vi "Receive Telemetry Packet.vi"(11 "UDP Network Connection in":refnum<k16>) -> (2 "Telemetry Packet":T1)   [LabVIEW 2015]
uses:
  Telemetry Packet Type.ctl
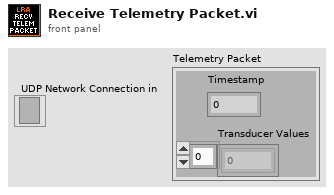
[diagram p1: front panel]
types:
  T1 = typedef "Telemetry Packet Type.ctl" = cluster{"Timestamp\n":u32, "Transducer Values":dbl[]}
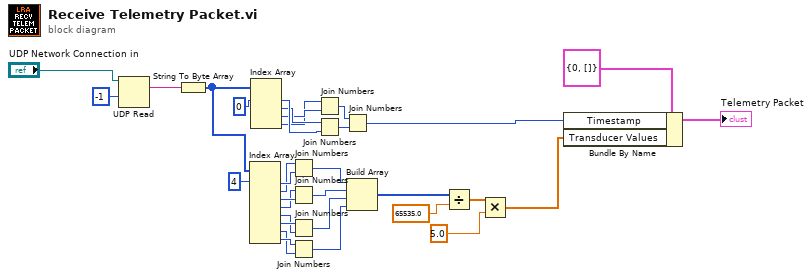
[diagram p0: block diagram]
diagram:
  n1 = UDP Read(connection ID="UDP Network Connection in", timeout ms (25000)=-1) -> (data out=w30:string)  [unwired: 2 in, 4 out]
  n2 = String To Byte Array(string=w30) -> (unsigned byte array=w19:u8[])
  n3 = Index Array(array=w19, index #1=4 ("index")) -> (element #1=w17:u8, element #2=w16:u8, element #3=w15:u8, element #4=w14:u8, element #5=w11:u8, element #6=w13:u8, element #7=w10:u8, element #8=w12:u8)  [unwired: 7 in]
  n4 = Index Array(array=w19, index #1=0 ("index")) -> (element #1=w26:u8, element #2=w25:u8, element #3=w24:u8, element #4=w23:u8)  [unwired: 3 in]
  n5 = Join Numbers(hi=w16, lo=w17) -> ((hi.lo)=w6:u16)
  n6 = Join Numbers(hi=w14, lo=w15) -> ((hi.lo)=w7:u16)
  n7 = Join Numbers(hi=w13, lo=w11) -> ((hi.lo)=w8:u16)
  n8 = Join Numbers(hi=w12, lo=w10) -> ((hi.lo)=w9:u16)
  n9 = Join Numbers(hi=w23, lo=w24) -> ((hi.lo)=w21:u16)
  n10 = Join Numbers(hi=w25, lo=w26) -> ((hi.lo)=w22:u16)
  n11 = Join Numbers(hi=w21, lo=w22) -> ((hi.lo)=w20:u32)
  n12 = Build Array(w6, w7, w8, w9) -> (w5:u16[])
  n13 = Divide(x=w5, y=65535.0) -> (x/y=w3:dbl[])
  n14 = Multiply(x=w3, y=5.0) -> (x*y=w1:dbl[])
  n15 = Bundle By Name(cluster=T1 {"Timestamp\n"=0, "Transducer Values"=[]}, "Timestamp"=w20, "Transducer Values"=w1) -> (→"Telemetry Packet":T1)
